vi "D2SParser - Private - Helper - Read Byte.vi"(8 "error in (no error)":errorcluster, 10 "Position":i64, 11 "D2SParser in":refnum<class "D2SParser.lvclass">) -> (0 "error out":errorcluster, 2 "byte":u8, 3 "D2SParser out":refnum<class "D2SParser.lvclass">)   [LabVIEW 2015, in "D2SParser.lvclass"]
uses:
  D2SParser.lvclass
  D2SParser.lvclass/D2SParser.ctl
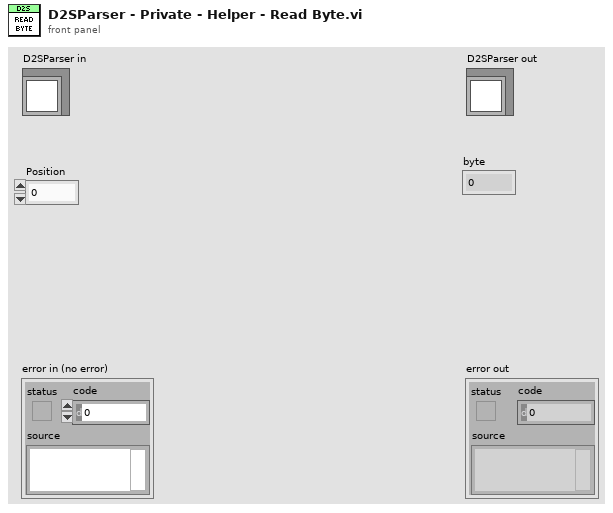
[diagram p1: front panel]
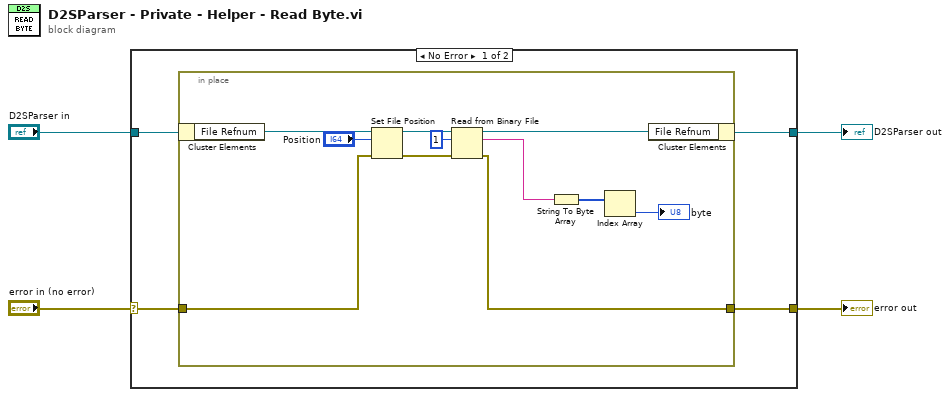
[diagram p0: block diagram]
diagram:
  n1 = case shown="No Error" "error in (no error)" {
    selector: "error in (no error)" -> [w7 w21]
    tunnel: [w6 w21] -> w3
    tunnel: [w5 w20] -> w1
    tunnel: "D2SParser in" -> [w8 w20]
    frame No Error {
      n2 = in-place {
        in-place-border: w7 -> [w14]
        in-place-border: [w10] -> w6
        n3 = in-place-cluster #1(w8) -> ("File Refnum"=w16:refnum<file>)
        n4 = Set File Position(offset (in bytes) (0)="Position", refnum=w16, error in=w14) -> (refnum out=w17:refnum<file>, error out=w18:errorcluster)  [unwired: 1 in]
        n5 = Read from Binary File(8:w18, 10:1 ("count (1)"), 11:w17) -> (0:w10:errorcluster, 2:w9:string, 3:w15:refnum<file>)  [unwired: 3 in, 1 out]
        n6 = String To Byte Array(string=w9) -> (unsigned byte array=w11:u8[])
        n7 = Index Array(array=w11) -> (element=→"byte":u8)  [unwired: 1 in]
        n8 = in-place-cluster #1("File Refnum"=w15) -> (w5:refnum<class "D2SParser.lvclass">)
      }
    }
    frame Error {
    }
  }
  "error out" <- w3
  "D2SParser out" <- w1
